vi "Add Style.vi"(8 "error in (no error)":errorcluster, 9 "Value":string, 10 "Style":string, 11 "Nav Route in":refnum<class "Nav Route.lvclass">) -> (0 "error out":errorcluster, 3 "Nav Route out":refnum<class "Nav Route.lvclass">)   [LabVIEW 2020, in "Volatus.lvlib" / "Nav Route.lvclass"]
uses:
  Nav Route.lvclass
  Nav Route.lvclass/Nav Route.ctl
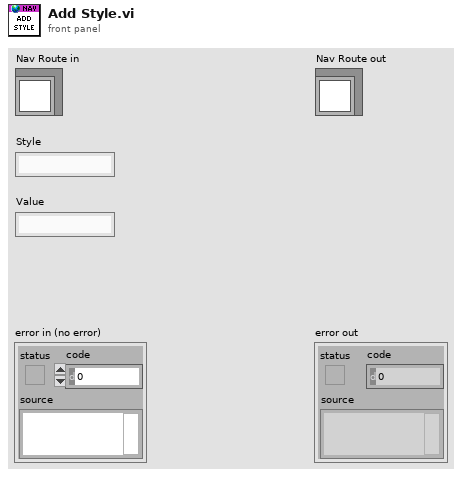
[diagram p1: front panel]
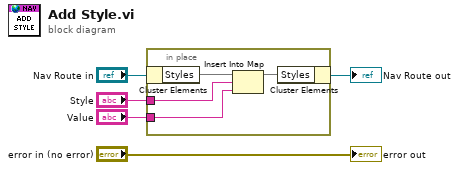
[diagram p0: block diagram]
diagram:
  n1 = in-place {
    in-place-border: "Style" -> [w8]
    in-place-border: "Value" -> [w7]
    n2 = in-place-cluster #1("Nav Route in") -> ("Styles"=w9:map{string, string})
    n3 = Insert Into Map(map in=w9, key=w8, value=w7) -> (map out=w6:map{string, string})  [unwired: 2 out]
    n4 = in-place-cluster #1("Styles"=w6) -> (→"Nav Route out":refnum<class "Nav Route.lvclass">)
  }
  "error out" <- "error in (no error)"
